vi "test adaptive FF 4.vi"() -> ()   [LabVIEW 2018]
uses:
  FPGA/Feed forward/FeedForwardProcessingState.ctl
  FPGA/Filters/biquad coefficients.ctl
  <vilib>/Utility/error.llb/Clear Errors.vi
  <vilib>/rvi/Emulation/niFpgaSctlEmulationGetInTimedLoop.vi
  <vilib>/rvi/Memory/Memory_Emulation/nirvimemoryFastEmulation.vi
  <vilib>/rvi/Memory/Memory_Emulation/nirvimemoryEmulation.vi
  <vilib>/rvi/Emulation/niFpgaEmulationIsFPGAContextNoSignature.vi
  <vilib>/rvi/DataTransferAndStorage/Container/Common/niFpgaContainerGetUniqueNameForEmu.vi
  <vilib>/rvi/Emulation/niFpgaProcessEmulError.vi
  <vilib>/rvi/errors/nirviReportUnexpectedCaseInternalError (U32).vi
  <vilib>/rvi/Memory/Memory_Emulation/niFpgaMemoryEmulationCacheClearOnFirstRun.vi
  <vilib>/rvi/Memory/Memory_Emulation/nirvimemoryEmulationManagerCache_MakeExclusive.vi
  <vilib>/rvi/Memory/Memory_Emulation/niFpgaMemoryEmulationValidateCache.vi
  <vilib>/rvi/Memory/Memory_Emulation/nirvimemoryEmulationManagerCache_InsertValue.vi
  <vilib>/rvi/Memory/Memory_Emulation/nirvimemoryEmulationManagerCache_ReleaseExclusive.vi
  <vilib>/rvi/Memory/Memory_Emulation/nirvimemoryEmulationManagerCache_GetValue.vi
  <vilib>/rvi/Memory/Memory_Emulation/nirvimemoryEmulationManagerCache_SetValue.vi
  <instrlib>/_niInstr/Basic Elements/v1/FPGA/Private/Count Down U8.vi
  <vilib>/rvi/DataTransferAndStorage/Container/XNode/niFpgaContainer.xnode
  <vilib>/rvi/DataTransferAndStorage/Register/Emulation/niFpgaRegisterEmulation.vi
  <instrlib>/_niInstr/Basic Elements/v1/FPGA/niInstr Basic Elements v1 FPGA.lvlib
panel:
  out "Waveform Graph 2":dbl[][](graph)
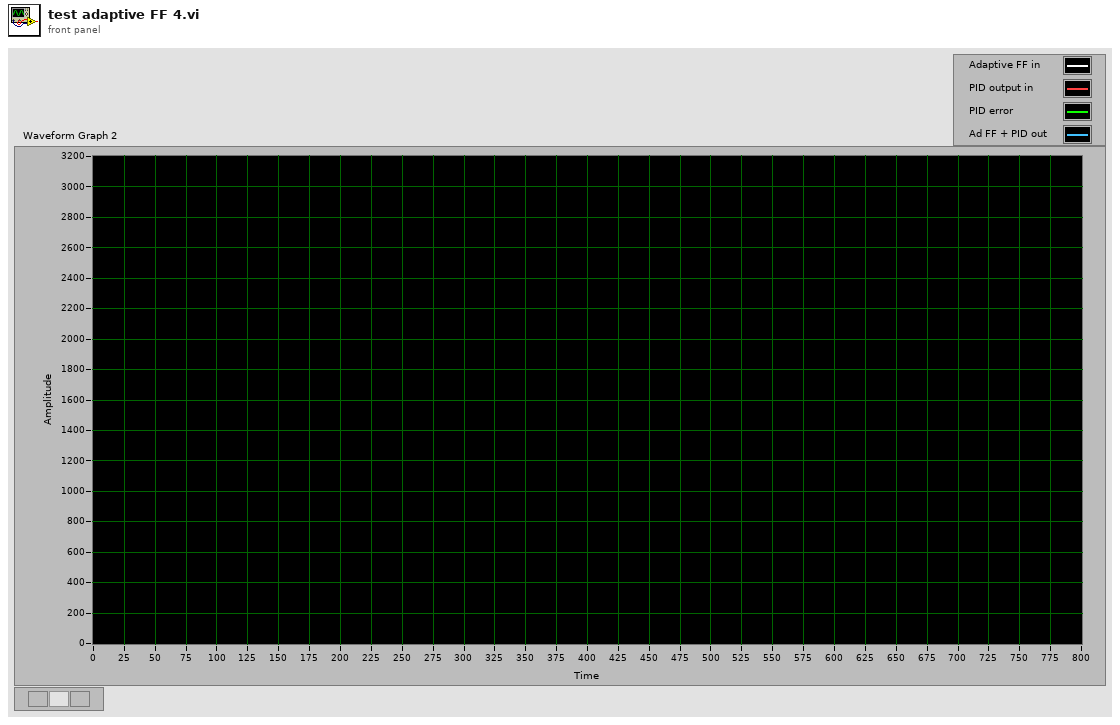
[diagram p1: front panel]
types:
  T1 = typedef "biquad coefficients.ctl" = cluster{"b0":fxp<+/-,32,2>, "b1":fxp<+/-,32,2>, "b2":fxp<+/-,32,2>, "-a1":fxp<+/-,32,2>, "-a2":fxp<+/-,32,2>}
  T2 = typedef "FeedForwardProcessingState.ctl" = enum16{"Wait for trigger", "Processing", "Filtering", "Process complete", "Read FF", "Clear FF", "Wait for reset"}
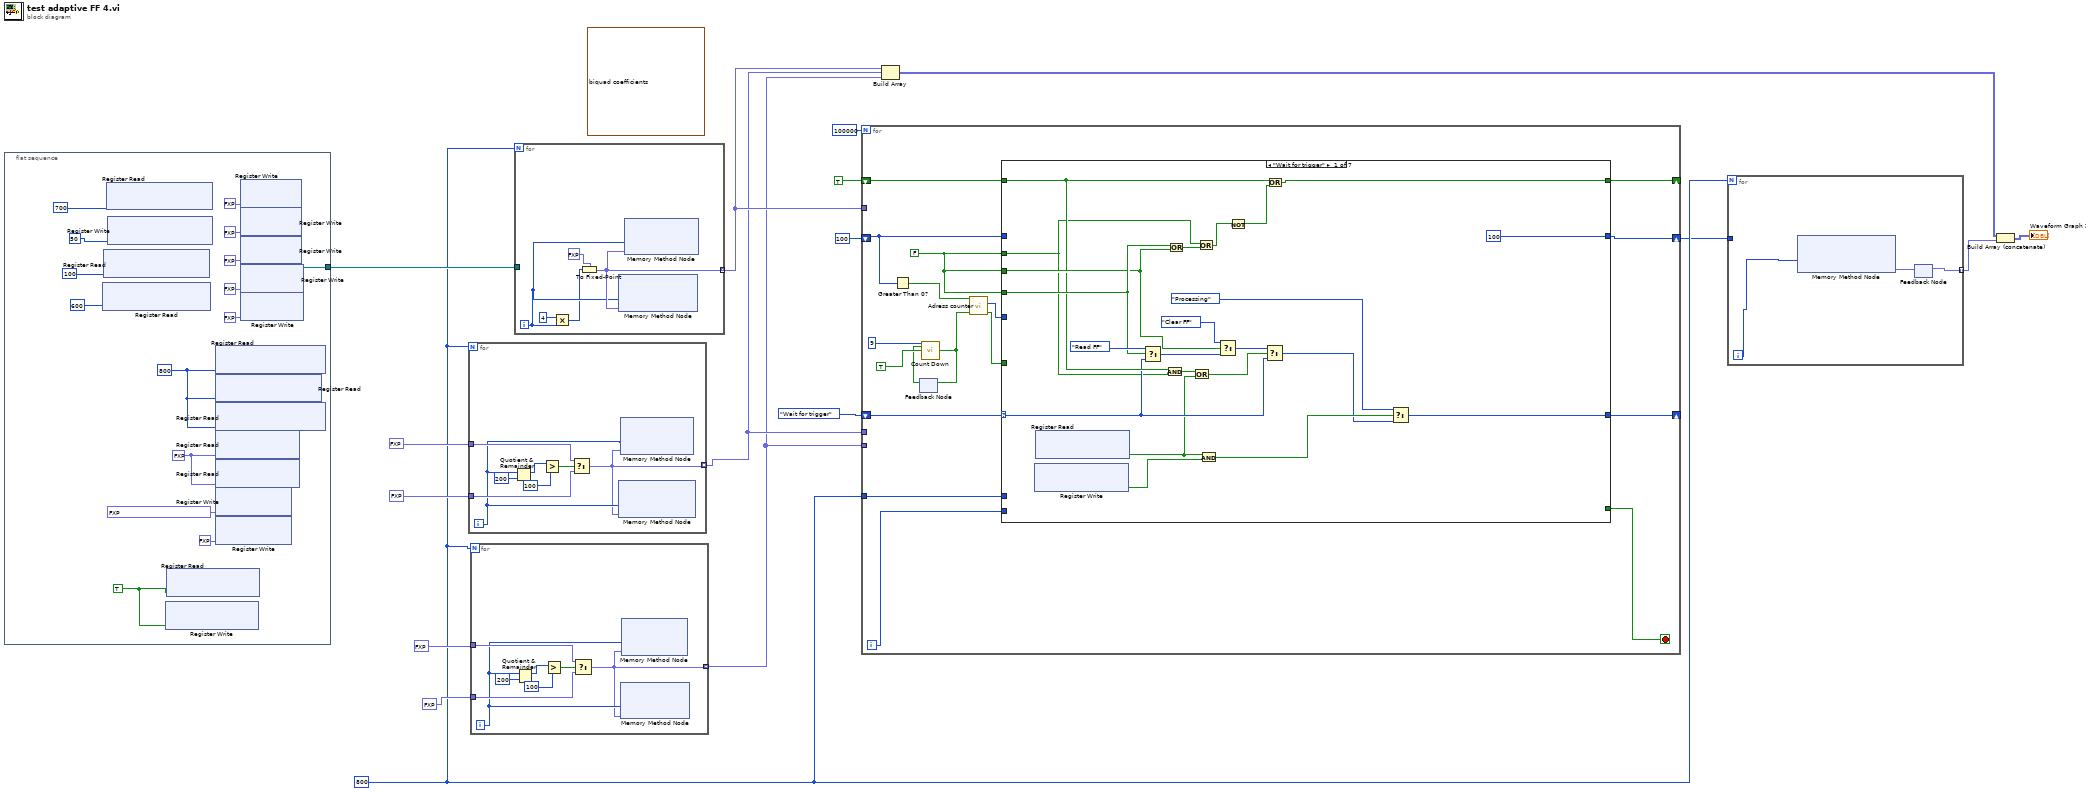
[diagram p0: block diagram]
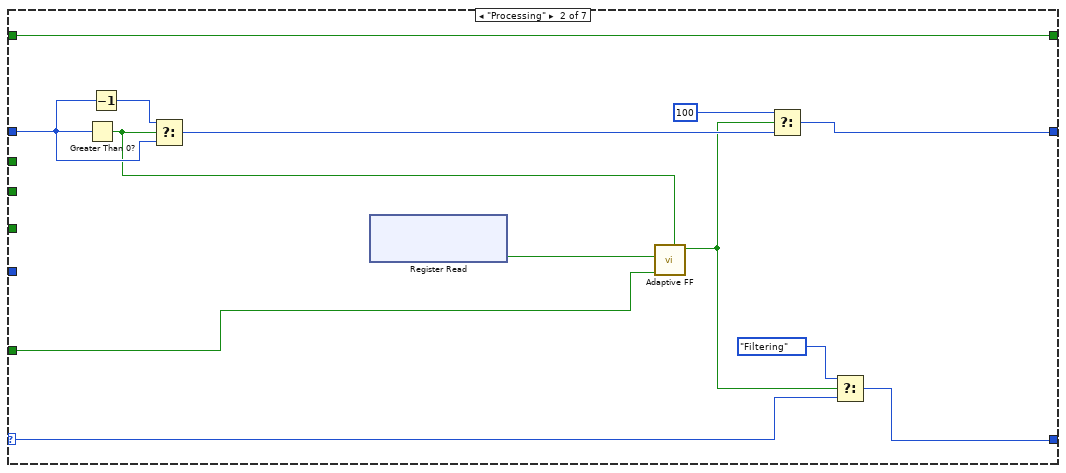
[diagram p2: hidden frame]
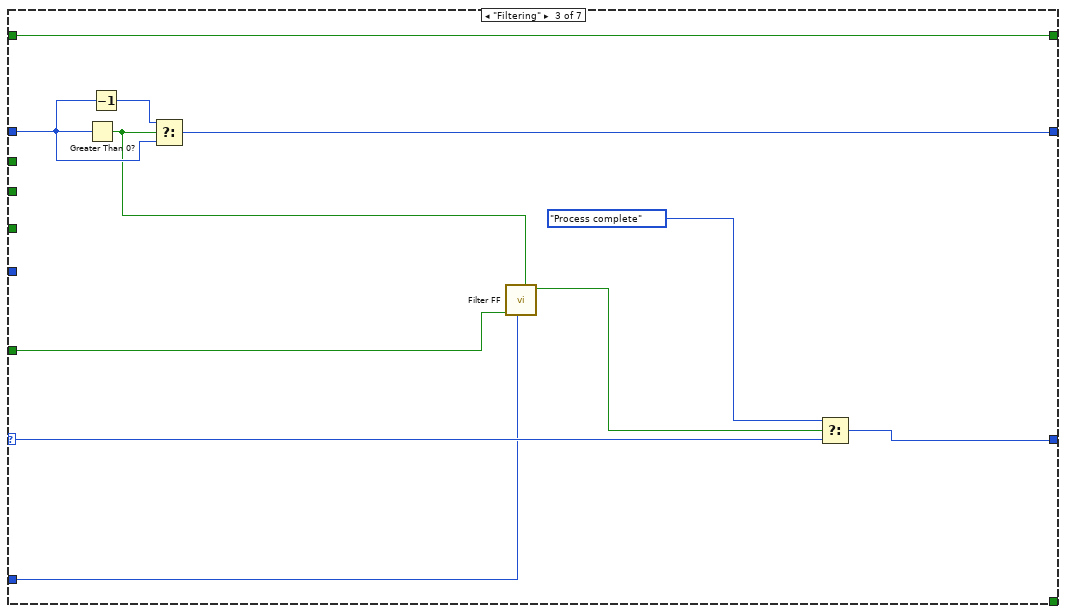
[diagram p3: hidden frame]
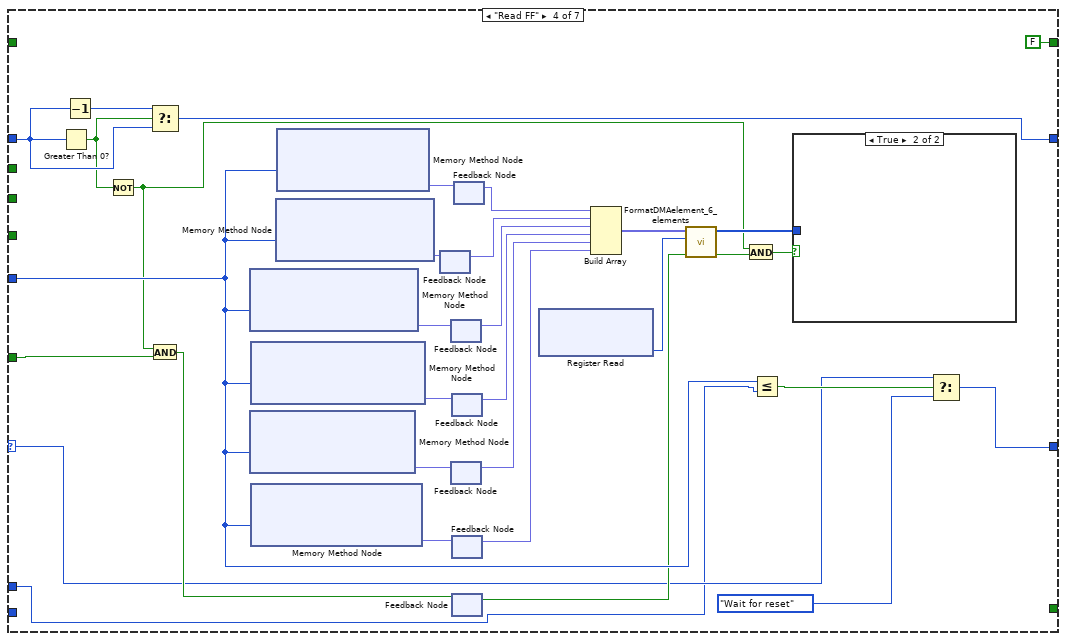
[diagram p4: hidden frame]
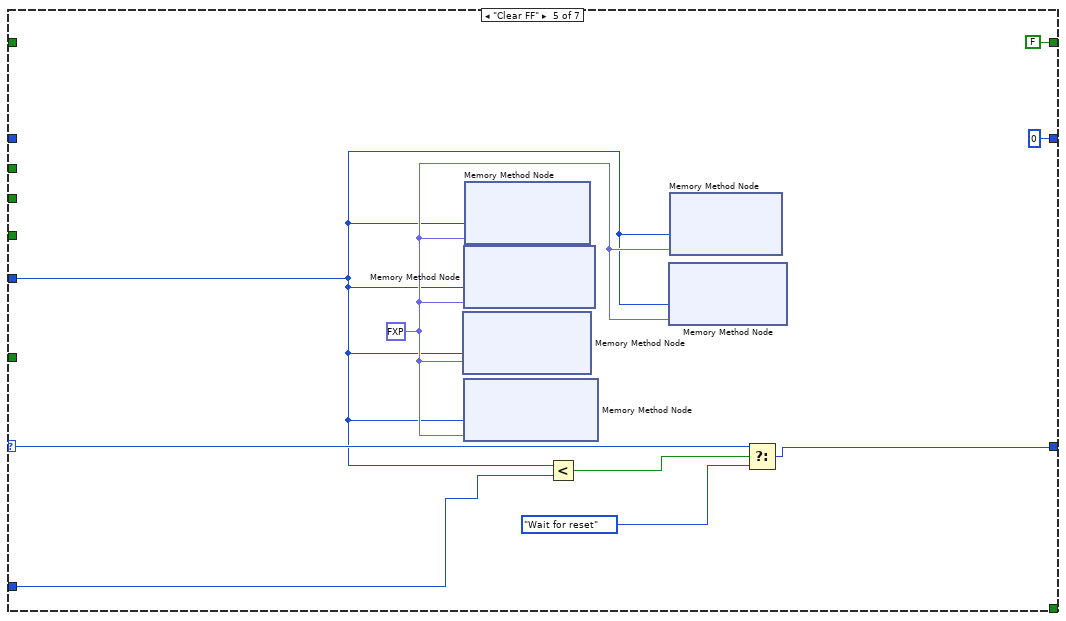
[diagram p6: hidden frame]
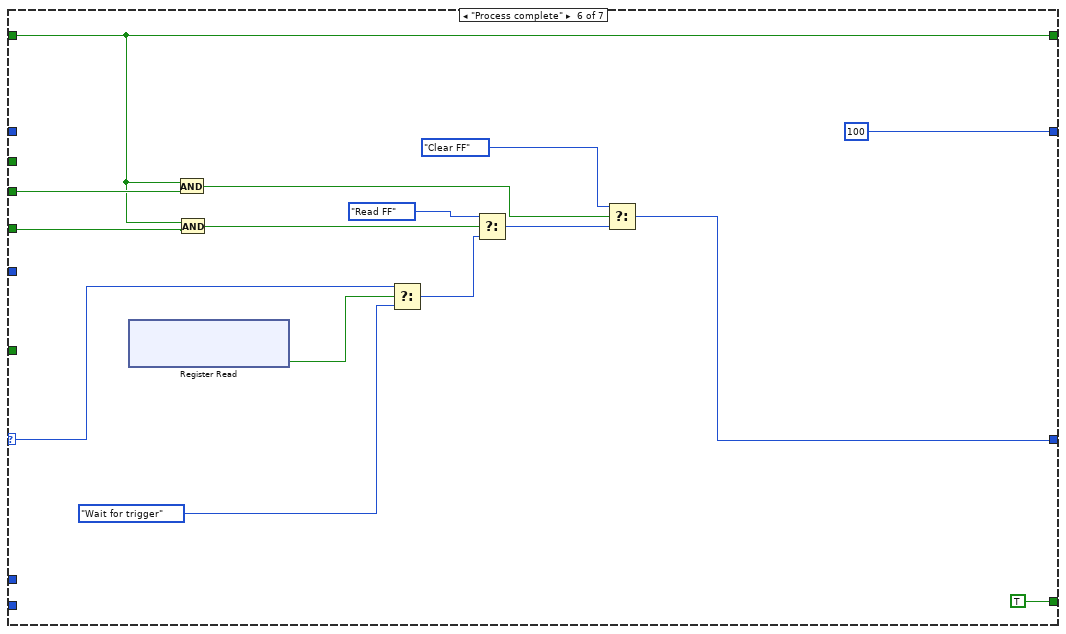
[diagram p7: hidden frame]
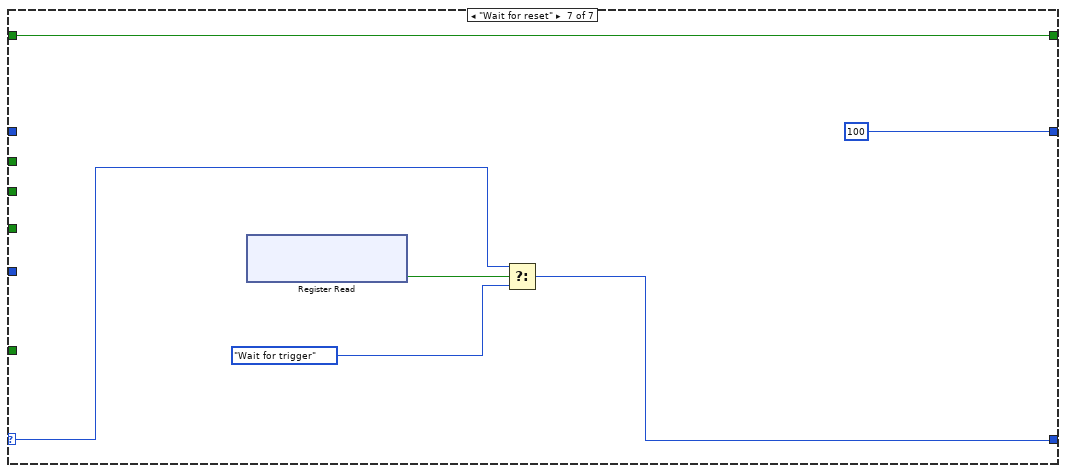
[diagram p8: hidden frame]
diagram:
  w3 = u32 800 ("Data")
  (unwired) T1 {"b0"=0.0038999998942017555, "b1"=0.007832200266420841, "b2"=0.0038999998942017555, "-a1"=1.8152999999001622, "-a2"=-0.8310000002384186} ("coefficients")
  n1 = flat-sequence {
    tunnel: [w27] -> w7
    frame #0 {
      w18 = TRUE ("Data")
      w25 = fxp<+/-,32,2> 0.5 ("Data")
      w26 = u32 800 ("Data")
      n2 = xnode "Register Read"("Data"=u32 600) -> ()  [unwired: 1 in, 1 out]
      n3 = xnode "Register Read"("Data"=u32 100) -> ()  [unwired: 1 in, 1 out]
      n4 = xnode "Register Read"("Data"=u32 700) -> ()  [unwired: 1 in, 1 out]
      n5 = xnode "Register Write"("Data"=u32 50) -> ()  [unwired: 1 in, 1 out]
      n6 = xnode ("Register Write")("Data"=w18) -> ()  [unwired: 1 in, 1 out]
      n7 = xnode ("Register Read")("Data"=w18) -> ()  [unwired: 1 in, 1 out]
      n8 = xnode ("Register Read")("Data"=w26) -> ()  [unwired: 1 in, 1 out]
      n9 = xnode "Register Read"("Data"=w26) -> ()  [unwired: 1 in, 1 out]
      n10 = xnode ("Register Read")("Data"=w26) -> ()  [unwired: 1 in, 1 out]
      n11 = xnode ("Register Read")("Data"=w25) -> ()  [unwired: 1 in, 1 out]
      n12 = xnode ("Register Read")("Data"=w25) -> ()  [unwired: 1 in, 1 out]
      n13 = xnode "Register Write"("Data"=fxp<+/-,32,4> 0.8999999985098839) -> ()  [unwired: 1 in, 1 out]
      n14 = xnode "Register Write"("Data"=fxp<+/-,32,17> 0.0) -> ()  [unwired: 1 in, 1 out]
      n15 = xnode "Register Write"("Data"=fxp<+/-,32,2> 1.0) -> ()  [unwired: 1 in, 1 out]
      n16 = xnode "Register Write"("Data"=fxp<+/-,32,2> 0.0) -> ()  [unwired: 1 in, 1 out]
      n17 = xnode "Register Write"("Data"=fxp<+/-,32,2> 0.0) -> ()  [unwired: 1 in, 1 out]
      n18 = xnode "Register Write"("Data"=fxp<+/-,32,2> 0.0) -> ("Register Out"=w27:refnum<k21>)  [unwired: 1 in]
      n19 = xnode "Register Write"("Data"=fxp<+/-,32,2> 0.0) -> ()  [unwired: 1 in, 1 out]
    }
  }
  n20 = for {
    N: w3 -> [_]
    tunnel: fxp<+/-,32,14> 100.0 ("Data") -> [w36]
    tunnel: fxp<+/-,32,14> 500.0 ("Data") -> [w35]
    tunnel: [w33] -> w10 mode=indexing
    i -> [w34]
    n21 = Quotient & Remainder(x=w34, y=200) -> (x-y*floor(x/y)=w39:i32)  [unwired: 1 out]
    n22 = Greater?(x=w39, y=100) -> (0:w37:bool)
    n23 = Select(t=w36, s=w37, f=w35) -> (s? t:f=w33:fxp<+/-,32,14>)
    n24 = xnode ("Memory Method Node")("Address"=w34, "Data"=w33) -> ()  [unwired: 1 in, 1 out]
    n25 = xnode ("Memory Method Node")("Address"=w34, "Data"=w33) -> ()  [unwired: 1 in, 1 out]
  }
  n26 = for {
    N: w3 -> [_]
    tunnel: fxp<+/-,32,14> 800.0 ("Data") -> [w45]
    tunnel: fxp<+/-,32,14> 400.0 ("Data") -> [w44]
    tunnel: [w42] -> w4 mode=indexing
    i -> [w43]
    n27 = Quotient & Remainder(x=w43, y=200) -> (x-y*floor(x/y)=w47:i32)  [unwired: 1 out]
    n28 = Greater?(x=w47, y=100) -> (0:w41:bool)
    n29 = Select(t=w45, s=w41, f=w44) -> (s? t:f=w42:fxp<+/-,32,14>)
    n30 = xnode ("Memory Method Node")("Address"=w43, "Data"=w42) -> ()  [unwired: 1 in, 1 out]
    n31 = xnode ("Memory Method Node")("Address"=w43, "Data"=w42) -> ()  [unwired: 1 in, 1 out]
  }
  n32 = for {
    N: w3 -> [_]
    tunnel: [w52] -> w11 mode=indexing
    tunnel: w7 -> [_]
    i -> [w50]
    n33 = Multiply(x=4, y=w50) -> (x*y=w49:i32)
    n34 = To Fixed-Point(fixed-point type=fxp<+/-,32,14> 0.0 ("Data"), number=w49) -> (fixed-point=w52:fxp<+/-,32,14>)
    n35 = xnode ("Memory Method Node")("Address"=w50, "Data"=w52) -> ()  [unwired: 1 in, 1 out]
    n36 = xnode ("Memory Method Node")("Address"=w50, "Data"=w52) -> ()  [unwired: 1 in, 1 out]
  }
  n37 = for {
    N: 100000 -> [_]
    shift-right: [w61] -> w1
    shift-left: u8 100 ("s? t:f") -> [w58]
    tunnel: w11 -> [_]
    tunnel: w10 -> [_]
    shift-right: [w63] -> _
    shift-left: FeedForwardProcessingState."Wait for trigger" ("Processing state") -> [w64]
    tunnel: w3 -> [w56]
    tunnel: w4 -> [_]
    shift-right: [w62] -> _
    shift-left: TRUE -> [w67]
    i -> [w54]
    stop <- w55 stop-if-true
    w66 = FALSE ("FF buffers manual")
    n38 = Greater Than 0?(x=w58) -> (x > 0?=w65:bool)
    n39 = feedback #1() -> (w68:bool)  [unwired: 1 in]
    n40 = call-poly <instrlib>:"Count Down.vi"("count in"=u8 9, "load"=w68, "decrement"=TRUE) -> ("terminal count"=w57:bool)  [unwired: 11 in, 1 out]
    n41 = feedback-in #1(w57) -> ()
    n42 = call "Adress counter.vi"("input valid"=w57, "Reset"=w65) -> ("output valid"=w60:bool, "Address"=w59:u32)  [unwired: 8 in]
    n43 = case shown="\"Wait for trigger\"" w64 {
      selector: w64 -> [w80 w98 w112 w124 w155 w167 w174]
      tunnel: w60 -> [_ w95 w109 w127 _ _ _]
      tunnel: [w76 w96 w110 w122 w152 w165 w178] -> w63
      tunnel: w58 -> [_ w104 w115 w130 _ _ _]
      tunnel: [u8 100 ("unsigned 8bit integer") w100 w108 w129 u8 0 ("unsigned 8bit integer") u8 100 ("unsigned 8bit integer") u8 100 ("unsigned 8bit integer")] -> w61
      tunnel: w66 -> [w79 _ _ _ _ _ _]
      tunnel: w66 -> [w85 _ _ _ _ w163 _]
      tunnel: w66 -> [w86 _ _ _ _ w160 _]
      tunnel: w59 -> [_ _ _ w132 w154 _ _]
      tunnel: w67 -> [w84 w93 w107 _ _ w161 w173]
      tunnel: [w81 w93 w107 FALSE ("decrement") FALSE ("decrement") w161 w173] -> w62
      tunnel: w56 -> [_ _ w106 w117 w149 _ _]
      tunnel: [_ _ _ _ _ TRUE _] -> w55
      tunnel: w54 -> [_ _ _ _ _ _ _]
      frame "Wait for trigger" {
        n44 = xnode ("Register Write")() -> ("Data"=w78:bool)  [unwired: 1 in, 1 out]
        n45 = xnode ("Register Read")() -> ("Data"=w72:bool)  [unwired: 1 in, 1 out]
        n46 = Select(t=FeedForwardProcessingState."Read FF" ("Processing state"), s=w86, f=w80) -> (s? t:f=w91:T2)
        n47 = And(x=w84, y=w79) -> (x .and. y?=w73:bool)
        n48 = Or(x=w86, y=w85) -> (x .or. y?=w87:bool)
        n49 = Or(x=w73, y=w72) -> (x .or. y?=w71:bool)
        n50 = Or(x=w79, y=w87) -> (x .or. y?=w83:bool)
        n51 = And(x=w72, y=w78) -> (x .and. y?=w77:bool)
        n52 = Select(t=FeedForwardProcessingState."Clear FF" ("Processing state"), s=w85, f=w91) -> (s? t:f=w88:T2)
        n53 = Not(x=w83) -> (.not. x?=w82:bool)
        n54 = Select(t=w88, s=w71, f=w80) -> (s? t:f=w74:T2)
        n55 = Or(x=w84, y=w82) -> (x .or. y?=w81:bool)
        n56 = Select(t=FeedForwardProcessingState."Processing" ("Processing state"), s=w77, f=w74) -> (s? t:f=w76:T2)
      }
      frame "Processing" {
        n57 = Greater Than 0?(x=w104) -> (x > 0?=w103:bool)
        n58 = Decrement(x=w104) -> (x-1=w105:u8)
        n59 = Select(t=w105, s=w103, f=w104) -> (s? t:f=w101:u8)
        n60 = xnode ("Register Read")() -> ("Data"=w94:bool)  [unwired: 1 in, 1 out]
        n61 = call "Adaptive FF.vi"("Reset"=w103, "input valid"=w95, "Disable e(n)"=w94) -> ("done"=w99:bool)  [unwired: 7 in, 1 out]
        n62 = Select(t=u8 100 ("s? t:f"), s=w99, f=w101) -> (s? t:f=w100:u8)
        n63 = Select(t=FeedForwardProcessingState."Filtering", s=w99, f=w98) -> (s? t:f=w96:T2)
      }
      frame "Filtering" {
        n64 = Greater Than 0?(x=w115) -> (x > 0?=w114:bool)
        n65 = Decrement(x=w115) -> (x-1=w116:u8)
        n66 = Select(t=w116, s=w114, f=w115) -> (s? t:f=w108:u8)
        n67 = call "Filter FF.vi"("Reset"=w114, "Elements in buffer"=w106, "input valid"=w109) -> ("done"=w113:bool)  [unwired: 7 in, 1 out]
        n68 = Select(t=FeedForwardProcessingState."Process complete", s=w113, f=w112) -> (s? t:f=w110:T2)
      }
      frame "Read FF" {
        n69 = Greater Than 0?(x=w130) -> (x > 0?=w128:bool)
        n70 = Decrement(x=w130) -> (x-1=w131:u8)
        n71 = Not(x=w128) -> (.not. x?=w119:bool)
        n72 = Select(t=w131, s=w128, f=w130) -> (s? t:f=w129:u8)
        n73 = And(x=w119, y=w127) -> (x .and. y?=w126:bool)
        n74 = xnode ("Memory Method Node")("Address"=w132) -> ("Data"=w148:fxp<+/-,32,14>)  [unwired: 1 in, 1 out]
        n75 = xnode ("Memory Method Node")("Address"=w132) -> ("Data"=w143:fxp<+/-,32,14>)  [unwired: 1 in, 1 out]
        n76 = xnode ("Memory Method Node")("Address"=w132) -> ("Data"=w147:fxp<+/-,32,14>)  [unwired: 1 in, 1 out]
        n77 = xnode ("Memory Method Node")("Address"=w132) -> ("Data"=w142:fxp<+/-,32,14>)  [unwired: 1 in, 1 out]
        n78 = xnode ("Memory Method Node")("Address"=w132) -> ("Data"=w134:fxp<+/-,32,14>)  [unwired: 1 in, 1 out]
        n79 = xnode ("Memory Method Node")("Address"=w132) -> ("Data"=w136:fxp<+/-,32,14>)  [unwired: 1 in, 1 out]
        n80 = feedback #2() -> (w133:fxp<+/-,32,14>)  [unwired: 1 in]
        n81 = feedback-in #2(w134) -> ()
        n82 = feedback #3() -> (w146:fxp<+/-,32,14>)  [unwired: 1 in]
        n83 = feedback-in #3(w148) -> ()
        n84 = feedback #4() -> (w141:fxp<+/-,32,14>)  [unwired: 1 in]
        n85 = feedback-in #4(w143) -> ()
        n86 = feedback #5() -> (w145:fxp<+/-,32,14>)  [unwired: 1 in]
        n87 = feedback-in #5(w147) -> ()
        n88 = feedback #6() -> (w140:fxp<+/-,32,14>)  [unwired: 1 in]
        n89 = feedback-in #6(w142) -> ()
        n90 = feedback #7() -> (w125:bool)  [unwired: 1 in]
        n91 = feedback-in #7(w126) -> ()
        n92 = feedback #8() -> (w135:fxp<+/-,32,14>)  [unwired: 1 in]
        n93 = feedback-in #8(w136) -> ()
        n94 = xnode ("Register Read")() -> ("Data"=w138:u16)  [unwired: 1 in, 1 out]
        n95 = Build Array(w135, w133, w146, w145, w141, w140) -> (w139:fxp<+/-,32,14>[])
        n96 = call "FormatDMAelement_6_elements.vi"("valid in"=w125, "factor"=w138, "Data in"=w139) -> ("valid out"=w121:bool, "Values"=w137:u64[])  [unwired: 7 in]
        n97 = And(x=w119, y=w121) -> (x .and. y?=w120:bool)
        n98 = Less Or Equal?(x=w132, y=w117) -> (x <= y?=w144:bool)
        n99 = case shown="True" w120 {
          tunnel: w137 -> [_ _]
          frame False {
          }
          frame True {
          }
        }
        n100 = Select(t=w124, s=w144, f=FeedForwardProcessingState."Wait for reset" ("Processing state")) -> (s? t:f=w122:T2)
      }
      frame "Clear FF" {
        w157 = fxp<+/-,32,14> 0.0 ("Data")
        n101 = xnode ("Memory Method Node")("Address"=w154, "Data"=w157) -> ()  [unwired: 1 in, 1 out]
        n102 = xnode ("Memory Method Node")("Address"=w154, "Data"=w157) -> ()  [unwired: 1 in, 1 out]
        n103 = xnode ("Memory Method Node")("Address"=w154, "Data"=w157) -> ()  [unwired: 1 in, 1 out]
        n104 = xnode ("Memory Method Node")("Address"=w154, "Data"=w157) -> ()  [unwired: 1 in, 1 out]
        n105 = Less?(x=w154, y=w149) -> (x < y?=w156:bool)
        n106 = xnode ("Memory Method Node")("Address"=w154, "Data"=w157) -> ()  [unwired: 1 in, 1 out]
        n107 = xnode ("Memory Method Node")("Address"=w154, "Data"=w157) -> ()  [unwired: 1 in, 1 out]
        n108 = Select(t=w155, s=w156, f=FeedForwardProcessingState."Wait for reset" ("Processing state")) -> (s? t:f=w152:T2)
      }
      frame "Process complete" {
        n109 = xnode ("Register Read")() -> ("Data"=w170:bool)  [unwired: 1 in, 1 out]
        n110 = And(x=w161, y=w163) -> (x .and. y?=w162:bool)
        n111 = And(x=w161, y=w160) -> (x .and. y?=w159:bool)
        n112 = Select(t=w167, s=w170, f=FeedForwardProcessingState."Wait for trigger" ("Processing state")) -> (s? t:f=w166:T2)
        n113 = Select(t=FeedForwardProcessingState."Read FF" ("Processing state"), s=w159, f=w166) -> (s? t:f=w169:T2)
        n114 = Select(t=FeedForwardProcessingState."Clear FF" ("Processing state"), s=w162, f=w169) -> (s? t:f=w165:T2)
      }
      frame "Wait for reset" {
        n115 = xnode ("Register Read")() -> ("Data"=w176:bool)  [unwired: 1 in, 1 out]
        n116 = Select(t=w174, s=w176, f=FeedForwardProcessingState."Wait for trigger" ("Processing state")) -> (s? t:f=w178:T2)
      }
    }
  }
  n117 = Build Array(w11, w10, w4) -> (w9:fxp<+/-,32,14>[][])
  n118 = for {
    N: w3 -> [_]
    tunnel: [w181] -> w15 mode=indexing
    tunnel: w1 -> [_]
    i -> [w180]
    n119 = xnode ("Memory Method Node")("Address"=w180) -> ("Data"=w179:fxp<+/-,32,14>)  [unwired: 1 in, 1 out]
    n120 = feedback-in #9(w179) -> ()
    n121 = feedback #9() -> (w181:fxp<+/-,32,14>)  [unwired: 1 in]
  }
  n122 = Build Array (concatenate)(w9, w15) -> (→"Waveform Graph 2":fxp<+/-,32,14>[][])
